vi "Init.vi"() -> (3 "TEMPLATE Actor out":refnum<class "TEMPLATE Actor.lvclass">)   [LabVIEW 2025, in "_Template.lvlib" / "Templates.lvlib" / "TEMPLATE Actor.lvlib" / "TEMPLATE Actor.lvclass"]
uses:
  TEMPLATE Actor.lvclass
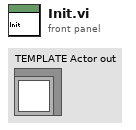
[diagram p1: front panel]
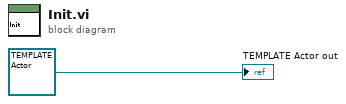
[diagram p0: block diagram]
diagram:
  "TEMPLATE Actor out" <- refnum<class "TEMPLATE Actor.lvclass"> refnum ("TEMPLATE Actor out")
